vi "Channel List.vi"(8 "Error In":errorcluster, 9 "Channel List":T1) -> (0 "Error Out":errorcluster, 1 "Channel String":string)   [LabVIEW 2016]
uses:
  Channel List.ctl
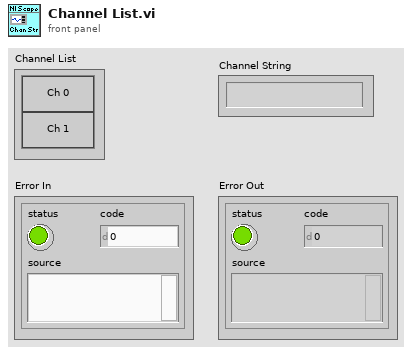
[diagram p1: front panel]
types:
  T1 = typedef "Channel List.ctl" = cluster{"Channel 0":bool, "Channel 1":bool}
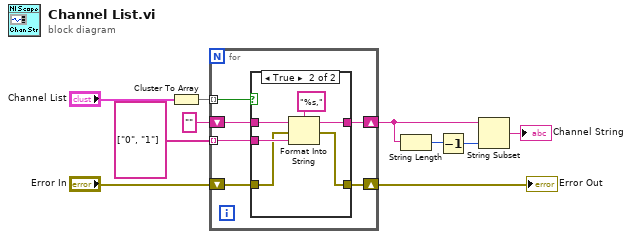
[diagram p0: block diagram]
diagram:
  n1 = Cluster To Array(cluster="Channel List") -> (array=w10:bool[])
  n2 = for {
    tunnel: w10 -> [w13] mode=indexing
    tunnel: string[] ["0", "1"] -> [w14] mode=indexing
    shift-right: [w16] -> w4
    shift-left: "" -> [w15]
    shift-right: [w12] -> w2
    shift-left: "Error In" -> [w11]
    n3 = case shown="True" w13 {
      tunnel: [w18 w22] -> w16
      tunnel: w15 -> [w18 w24]
      tunnel: w14 -> [_ w23]
      tunnel: [w17 w20] -> w12
      tunnel: w11 -> [w17 w19]
      frame False {
      }
      frame True {
        n4 = Format Into String(format string="%s,", initial string=w24, error in=w19, w23) -> (resulting string=w22:string, error out=w20:errorcluster)
      }
    }
  }
  "Error Out" <- w2
  n5 = String Length(string=w4) -> (length=w6:i32)
  n6 = Decrement(x=w6) -> (x-1=w5:i32)
  n7 = String Subset(string=w4, length (rest)=w5) -> (substring=→"Channel String":string)  [unwired: 1 in]
